vi "ConfigureInputsOutputs.vi"(0 "axis in":cluster{"keyHandle":u32, "nodeId":u16}={"keyHandle"=0, "nodeId"=1}, 5 "digital input configuration":T3={"digitalInputNumber"=1, "configuration"=15, "mask"=1, "polarity"=0, "executionMask"=1} {"executionMask" items=["Disabled", "Enabled"]; "polarity" items=["HighActive", "LowActive"]; "mask" items=["Disabled", "Enabled"]; "configuration" items=["Negative Limit Switch"=0, "Positive Limit Switch"=1, "Home Switch"=2, "Position Marker"=3, "Enable"=4, "General Purpose A"=15, "General Purpose B"=14, "General Purpose C"=13, "General Purpose D"=12, "General Purpose E"=11, "General Purpose F"=10, "General Purpose G"=9, "General Purpose H"=8]}, 7 "digital output configuration":T2={"digitalOutputNumber"=1, "configuration"=0, "state"=0, "mask"=0, "polarity"=0} {"polarity" items=["HighActive", "LowActive"]; "mask" items=["Disabled", "Enabled"]; "state" items=["Inactive", "Active"]; "configuration" items=["Ready"=0, "Position Compare"=1, "General Purpose A"=15, "General Purpose B"=14, "General Purpose C"=13, "General Purpose D"=12, "General Purpose E"=11, "General Purpose F"=10, "General Purpose G"=9, "General Purpose H"=8]}, 9 "analog input configuration":T1={"analogInputNumber"=1, "configuration"=15, "executionMask"=0} {"executionMask" items=["Disabled", "Enabled"]; "configuration" items=["current setpoint"=0, "velocity setpoint"=1, "position setpoint"=2, "general purpose A"=15, "general purpose B"=14, "general purpose C"=13, "general purpose D"=12, "general purpose E"=11]}, 11 "error in (no error)":errorcluster) -> (4 "axis out":cluster{"keyHandle":u32, "nodeId":u16}={"keyHandle"=0, "nodeId"=1}, 15 "error out":errorcluster)   [LabVIEW 2010]
doc: "<B>ConfigureInputsOutputs</B> writes the input and/or output configuration to the device."
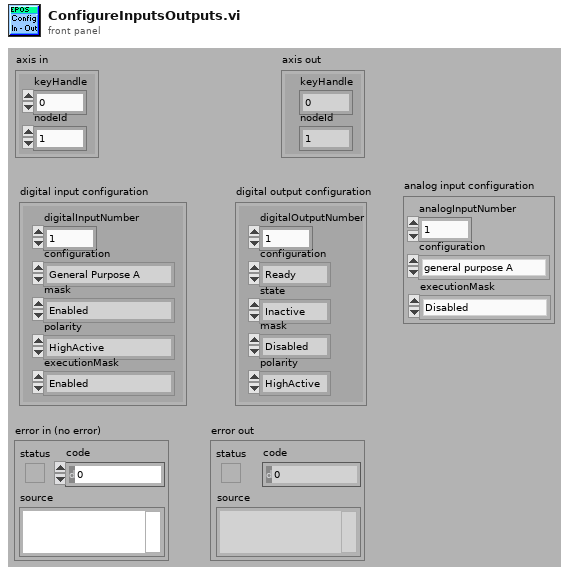
[diagram p1: front panel]
types:
  T1 = cluster{"analogInputNumber":u16, "configuration":u16, "executionMask":i32}
  T2 = cluster{"digitalOutputNumber":u16, "configuration":u16, "state":i32, "mask":i32, "polarity":i32}
  T3 = cluster{"digitalInputNumber":u16, "configuration":u16, "mask":i32, "polarity":i32, "executionMask":i32}
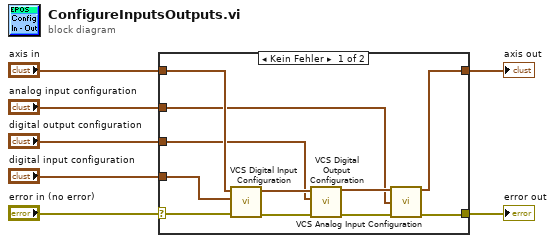
[diagram p0: block diagram]
diagram:
  n1 = case shown="Kein Fehler" "error in (no error)" {
    selector: "error in (no error)" -> [w18 w20]
    tunnel: [w15 w20] -> w6
    tunnel: [w14 w19] -> w5
    tunnel: "axis in" -> [w11 w19]
    tunnel: "digital input configuration" -> [w10 _]
    tunnel: "digital output configuration" -> [w9 _]
    tunnel: "analog input configuration" -> [w8 _]
    frame No Error {
      n2 = call "VCS Digital Input Configuration.vi"("error in (no error)"=w18, "input configuration"=w10, "axis in"=w11) -> ("error out"=w17:errorcluster, "axis out"=w12:cluster{"keyHandle":u32, "nodeId":u16})  [unwired: 7 in]
      n3 = call "VCS Digital Output Configuration.vi"("error in (no error)"=w17, "output configuration"=w9, "axis in"=w12) -> ("error out"=w16:errorcluster, "axis out"=w13:cluster{"keyHandle":u32, "nodeId":u16})  [unwired: 7 in]
      n4 = call "VCS Analog Input Configuration.vi"("axis in"=w13, "configuration"=w8, "error in (no error)"=w16) -> ("axis out"=w14:cluster{"keyHandle":u32, "nodeId":u16}, "error out"=w15:errorcluster)  [unwired: 11 in]
    }
    frame Error {
    }
  }
  "error out" <- w6
  "axis out" <- w5
